vi "Config-Get Keys.vi"(0 "configuration file path":path, 2 "section":string, 11 "error in (no error)":errorcluster) -> (4 "file path":path, 8 "key names":string[](array[string]), 15 "error out":errorcluster)   [LabVIEW 2020]
uses:
  <vilib>/Utility/config.llb/NI_LVConfig.lvlib
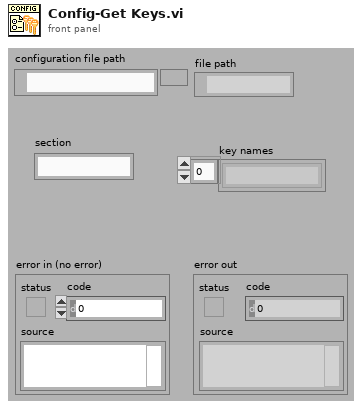
[diagram p1: front panel]
types:
  T1 = typedef "NI_LVConfig.lvlib/Config Data RefNum.ctl" = refnum<k1>
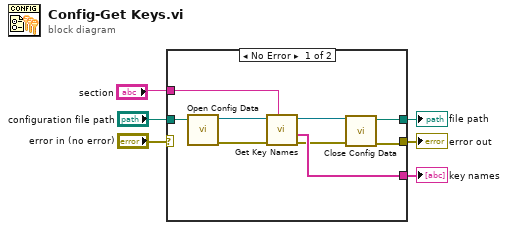
[diagram p0: block diagram]
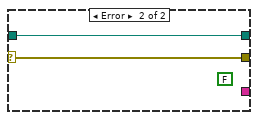
[diagram p2: hidden frame]
diagram:
  n1 = case shown="No Error" "error in (no error)" {
    selector: "error in (no error)" -> [_ w17]
    tunnel: [w15 w17] -> w6
    tunnel: "configuration file path" -> [w14 w16]
    tunnel: [w13 w16] -> w3
    tunnel: [w8 _] -> w2
    tunnel: "section" -> [w9 _]
    frame No Error {
      n2 = call <vilib>:"Open Config Data.vi"("configuration file path"=w14) -> ("error out"=w10:errorcluster, "refnum"=w12:T1)  [unwired: 8 in, 1 out]
      n3 = call <vilib>:"Get Key Names.vi"("section"=w9, "error in (no error)"=w10, "refnum"=w12) -> ("error out"=w7:errorcluster, "key names"=w8:string[], "refnum out"=w11:T1)  [unwired: 5 in, 1 out]
      n4 = call <vilib>:"Close Config Data.vi"("error in (no error)"=w7, "refnum"=w11) -> ("error out"=w15:errorcluster, "file path"=w13:path)  [unwired: 8 in]
    }
    frame Error {
      (unwired) FALSE ("found?")
    }
  }
  "error out" <- w6
  "file path" <- w3
  "key names" <- w2
